vi "Begin.vi"(8 "error in":errorcluster) -> (0 "error out":errorcluster)   [LabVIEW 2018]
doc: "Called before other user functions, this VI can be used to open I/O refnums, load in file data, and do general program initialization. Notice that the <B>error out</B> terminal is simply used for data flow. Wiring it to other structures or subVIs ensures that this VI runs first."
uses:
  <vilib>/Rock Robotics/WPI/DriverStation/WPI_DriverStationRobotMode2.ctl
  <vilib>/Rock Robotics/WPI/Joystick/WPI_JoystickDeviceEnum.ctl
  <vilib>/Rock Robotics/SystemInterfaces/DIO/FPGA_DIOPWMChannel.ctl
  <vilib>/Rock Robotics/WPI/Solenoid/WPI_SolenoidChannel.ctl
  <vilib>/Rock Robotics/WPI/Solenoid/WPI_SolenoidValue.ctl
  <vilib>/Rock Robotics/WPI/SafetyOutput/WPI_SafetyOutputConfigMenu.ctl
  Robot Global Data.vi
  <vilib>/Rock Robotics/WPI/RobotDrive/WPI_RobotDriveOpen4MotorWithExistingMotors.vi
  <vilib>/Rock Robotics/WPI/RobotDrive/WPI_RobotDriveOpen2MotorWithExistingMotors.vi
  <vilib>/Rock Robotics/WPI/MotorControl/WPI_MotorControlOpen SPARK.vi
  <vilib>/Rock Robotics/WPI/Solenoid/WPI_SolenoidOpenDouble.vi
  <vilib>/Rock Robotics/WPI/Solenoid/WPI_SolenoidSetEnum.vi
panel:
  in  "Power Distribution Panel (0)":u8
  in  "Clear Sticky Faults":bool=TRUE
  out "Current Faults":bool[](array[boolean])
  out "Battery Voltage Fault":bool
  out "Temperature Fault":bool
  out "Hardware Fault":bool
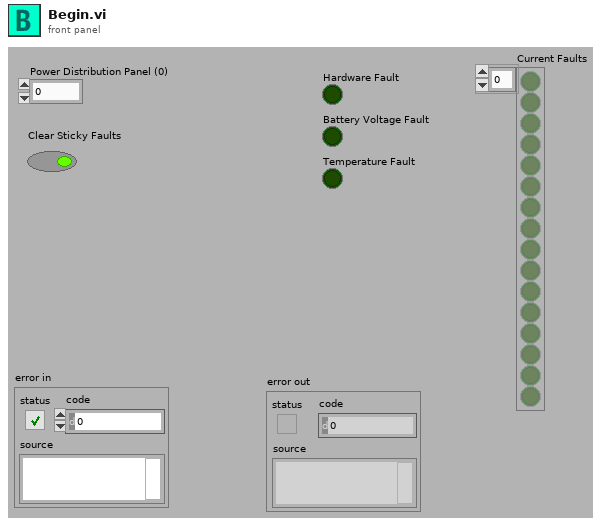
[diagram p1: front panel]
types:
  T1 = typedef "WPI_SafetyOutputConfigMenu.ctl" = enum16{"Enable", "Disable"}
  T2 = typedef "WPI_SolenoidValue.ctl" = enum16{"Off", "On", "Forward", "Reverse"}
  T3 = typedef "WPI_SolenoidChannel.ctl" = enum8{"Solenoid 0", "Solenoid 1", "Solenoid 2", "Solenoid 3", "Solenoid 4", "Solenoid 5", "Solenoid 6", "Solenoid 7", "Invalid"}
  T4 = typedef "FPGA_DIOPWMChannel.ctl" = enum8{"PWM 0", "PWM 1", "PWM 2", "PWM 3", "PWM 4", "PWM 5", "PWM 6", "PWM 7", "PWM 8", "PWM 9", "PWM MXP 0", "PWM MXP 1", "PWM MXP 2", "PWM MXP 3", "PWM MXP 4", "PWM MXP 5", "PWM MXP 6", "PWM MXP 7", "PWM MXP 8", "PWM MXP 9", "Invalid"}
  T5 = typedef "WPI_JoystickDeviceEnum.ctl" = enum16{"USB 0", "USB 1", "USB 2", "USB 3", "USB 4", "USB 5"}
  T6 = typedef "WPI_DriverStationRobotMode2.ctl" = enum16{"Autonomous Disabled", "Autonomous Enabled", "Teleop Disabled", "Teleop Enabled", "Disconnected", "Finish", "Test Disabled", "Test Enabled", "Emergency Stopped"}
  T7 = typedef "WPI_JoystickDevRef.ctl" = cluster{"Device":T5}
  T8 = typedef "WPI_MotorControlDeviceRef.ctl" = cluster{"DeviceStatus":errorcluster, "Type":T9, "PWM":cluster{"PWM Channel":T4, "DeadBand":T10}, "CAN":cluster{"Device Number":u8, "SetOutput VI Ref":variant, "GetOutput VI Ref":variant, "Enable VI Ref":variant, "Disable VI Ref":variant, "Data":variant}, "Invert":bool, "DIO PWM":cluster{"PWM \"Enable\" Channel":T4, "DIOChannel":T11, "PWM Rate":dbl}}
  T9 = typedef "WPI_MotorControlType.ctl" = enum16{"PWM", "CAN", "DIO PWM"}
  T10 = typedef "WPI_PWMDeadband.ctl" = cluster{"Name":string, "maxPositivePwm":i32, "minPositivePwm":i32, "centerPwm":i32, "maxNegativePwm":i32, "minNegativePwm":i32, "angularRange":u16}
  T11 = typedef "FPGA_DIOChannel.ctl" = enum8{"DIO 0", "DIO 1", "DIO 2", "DIO 3", "DIO 4", "DIO 5", "DIO 6", "DIO 7", "DIO 8", "DIO 9", "DIO MXP 0", "DIO MXP 1", "DIO MXP 2", "DIO MXP 3", "DIO MXP 4", "DIO MXP 5", "DIO MXP 6", "DIO MXP 7", "DIO MXP 8", "DIO MXP 9", "DIO MXP 10", "DIO MXP 11", "DIO MXP 12", "DIO MXP 13", "DIO MXP 14", "DIO MXP 15", "SPI Port CS1", "SPI Port CS2", "SPI Port CS3", "SPI Port MISO", "SPI Port MOSI", "Invalid"}
  T12 = typedef "WPI_RobotDriveDevRef.ctl" = cluster{"DevStatus":errorcluster, "Motors[]":T8[], "Square Inputs":bool, "Max Output":dbl}
  T13 = typedef "WPI_SolenoidDevRef.ctl" = cluster{"DevStatus":errorcluster, "Pneumatics Control Module":u8, "Forward Solenoid Channel":T3, "Reverse Solenoid Channel":T3}
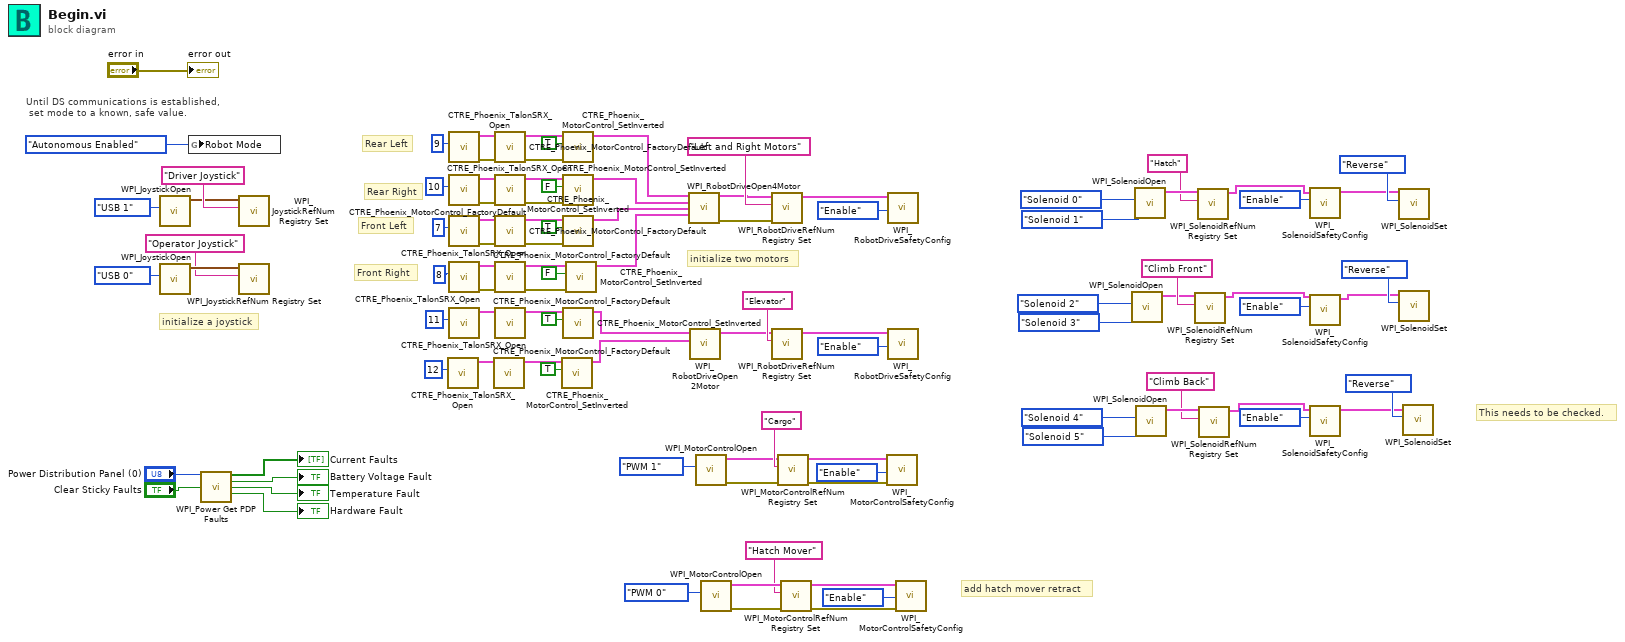
[diagram p0: block diagram]
diagram:
  # "This needs to be checked."
  # "add hatch mover retract"
  # "Front Right"
  # "Front Left"
  # "Rear Right"
  # "Rear Left"
  # "initialize two motors"
  # "initialize a joystick"
  # "Until DS communications is established,\n set mode to a known, safe value."
  n1 = call <vilib>:"WPI_JoystickOpen.vi"("JoystickDevice"=WPI_JoystickDeviceEnum."USB 1") -> ("JoystickDevRef"=w19:T7)  [unwired: 10 in]
  n2 = call <vilib>:"WPI_JoystickOpen.vi"("JoystickDevice"=WPI_JoystickDeviceEnum."USB 0") -> ("JoystickDevRef"=w16:T7)  [unwired: 10 in]
  n3 = global write "Robot Global Data.vi" "Robot Mode"(WPI_DriverStationRobotMode2."Autonomous Enabled" ("Robot Mode")) -> ()
  n4 = call <vilib>:"WPI_Power Get PDP Faults.vi"("Power Distribution Panel (0)"="Power Distribution Panel (0)", "Clear Sticky Faults"="Clear Sticky Faults") -> ("Current Faults"=→"Current Faults":bool[], "Battery Voltage Fault"=→"Battery Voltage Fault":bool, "Temperature Fault"=→"Temperature Fault":bool, "Hardware Fault"=→"Hardware Fault":bool)  [unwired: 9 in, 1 out]
  n5 = call <vilib>:"WPI_JoystickRefNum Registry Set.vi"("refnum name"="Driver Joystick", "JoystickDevRef"=w19) -> ()  [unwired: 8 in, 2 out]
  n6 = call <vilib>:"WPI_JoystickRefNum Registry Set.vi"("refnum name"="Operator Joystick", "JoystickDevRef"=w16) -> ()  [unwired: 8 in, 2 out]
  n7 = call <vilib>:"CTRE_Phoenix_TalonSRX_Open.vi"("Device Number"=u8 12) -> ("CAN Talon SRX Ref"=w56:T8)  [unwired: 9 in, 1 out]
  n8 = call <vilib>:"CTRE_Phoenix_TalonSRX_Open.vi"("Device Number"=u8 9) -> ("error out"=w38:errorcluster, "CAN Talon SRX Ref"=w39:T8)  [unwired: 9 in]
  n9 = call <vilib>:"CTRE_Phoenix_TalonSRX_Open.vi"("Device Number"=u8 10) -> ("error out"=w40:errorcluster, "CAN Talon SRX Ref"=w41:T8)  [unwired: 9 in]
  n10 = call <vilib>:"CTRE_Phoenix_TalonSRX_Open.vi"("Device Number"=u8 7) -> ("error out"=w42:errorcluster, "CAN Talon SRX Ref"=w43:T8)  [unwired: 9 in]
  n11 = call <vilib>:"CTRE_Phoenix_TalonSRX_Open.vi"("Device Number"=u8 8) -> ("error out"=w44:errorcluster, "CAN Talon SRX Ref"=w45:T8)  [unwired: 9 in]
  n12 = call <vilib>:"CTRE_Phoenix_TalonSRX_Open.vi"("Device Number"=u8 11) -> ("CAN Talon SRX Ref"=w59:T8)  [unwired: 9 in, 1 out]
  n13 = call <vilib>:"CTRE_Phoenix_MotorControl_FactoryDefault.vi"("PhoenixMotorControlDevRef"=w56) -> ("PhoenixMotorControlDevRef"=w57:T8)  [unwired: 9 in, 1 out]
  n14 = call <vilib>:"CTRE_Phoenix_MotorControl_FactoryDefault.vi"("error in"=w38, "PhoenixMotorControlDevRef"=w39) -> ("error out"=w47:errorcluster, "PhoenixMotorControlDevRef"=w46:T8)  [unwired: 8 in]
  n15 = call <vilib>:"CTRE_Phoenix_MotorControl_FactoryDefault.vi"("error in"=w40, "PhoenixMotorControlDevRef"=w41) -> ("error out"=w49:errorcluster, "PhoenixMotorControlDevRef"=w48:T8)  [unwired: 8 in]
  n16 = call <vilib>:"CTRE_Phoenix_MotorControl_FactoryDefault.vi"("error in"=w42, "PhoenixMotorControlDevRef"=w43) -> ("error out"=w51:errorcluster, "PhoenixMotorControlDevRef"=w50:T8)  [unwired: 8 in]
  n17 = call <vilib>:"CTRE_Phoenix_MotorControl_FactoryDefault.vi"("error in"=w44, "PhoenixMotorControlDevRef"=w45) -> ("error out"=w53:errorcluster, "PhoenixMotorControlDevRef"=w52:T8)  [unwired: 8 in]
  n18 = call <vilib>:"CTRE_Phoenix_MotorControl_FactoryDefault.vi"("PhoenixMotorControlDevRef"=w59) -> ("PhoenixMotorControlDevRef"=w58:T8)  [unwired: 9 in, 1 out]
  n19 = call <vilib>:"CTRE_Phoenix_MotorControl_SetInverted.vi"("Invert?"=TRUE, "PhoenixMotorControlDevRef"=w57) -> ("PhoenixMotorControlDevRef"=w77:T8)  [unwired: 8 in, 1 out]
  n20 = call <vilib>:"CTRE_Phoenix_MotorControl_SetInverted.vi"("error in (no error)"=w47, "Invert?"=TRUE, "PhoenixMotorControlDevRef"=w46) -> ("PhoenixMotorControlDevRef"=w37:T8)  [unwired: 7 in, 1 out]
  n21 = call <vilib>:"CTRE_Phoenix_MotorControl_SetInverted.vi"("error in (no error)"=w49, "Invert?"=FALSE, "PhoenixMotorControlDevRef"=w48) -> ("PhoenixMotorControlDevRef"=w32:T8)  [unwired: 7 in, 1 out]
  n22 = call <vilib>:"CTRE_Phoenix_MotorControl_SetInverted.vi"("error in (no error)"=w51, "Invert?"=TRUE, "PhoenixMotorControlDevRef"=w50) -> ("PhoenixMotorControlDevRef"=w35:T8)  [unwired: 7 in, 1 out]
  n23 = call <vilib>:"CTRE_Phoenix_MotorControl_SetInverted.vi"("Invert?"=TRUE, "PhoenixMotorControlDevRef"=w58) -> ("PhoenixMotorControlDevRef"=w76:T8)  [unwired: 8 in, 1 out]
  n24 = call <vilib>:"CTRE_Phoenix_MotorControl_SetInverted.vi"("error in (no error)"=w53, "Invert?"=FALSE, "PhoenixMotorControlDevRef"=w52) -> ("PhoenixMotorControlDevRef"=w30:T8)  [unwired: 7 in, 1 out]
  n25 = call-poly <vilib>:"WPI_RobotDriveOpen4Motor.vi"("Rear Left Motor Dev Ref"=w37, "Rear Right Motor Dev Ref"=w32, "Front Left Motor Dev Ref"=w35, "Front Right Motor Dev Ref"=w30) -> ("RobotDriveDevRef"=w21:T12, "error out"=w23:errorcluster)  [unwired: 10 in]
  n26 = call-poly <vilib>:"WPI_RobotDriveOpen2Motor.vi"("Right Motor Dev Ref"=w77, "Left Motor Dev Ref"=w76) -> ("RobotDriveDevRef"=w80:T12)  [unwired: 8 in, 1 out]
  n27 = call-poly <vilib>:"WPI_MotorControlOpen.vi"("PWM Channel"=FPGA_DIOPWMChannel."PWM 1") -> ("error out"=w62:errorcluster, "MotorControlDeviceRef"=w63:T8)  [unwired: 9 in]
  n28 = call-poly <vilib>:"WPI_MotorControlOpen.vi"("PWM Channel"=FPGA_DIOPWMChannel."PWM 0") -> ("error out"=w75:errorcluster, "MotorControlDeviceRef"=w74:T8)  [unwired: 9 in]
  n29 = call <vilib>:"WPI_RobotDriveRefNum Registry Set.vi"("error in (no error)"=w23, "refnum name"="Left and Right Motors", "RobotDriveDevRef"=w21) -> ("RobotDriveDevRef"=w24:T12)  [unwired: 1 in, 7 out]
  n30 = call <vilib>:"WPI_RobotDriveRefNum Registry Set.vi"("refnum name"="Elevator", "RobotDriveDevRef"=w80) -> ("RobotDriveDevRef"=w79:T12)  [unwired: 2 in, 7 out]
  n31 = call <vilib>:"WPI_MotorControlRefNum Registry Set.vi"("error in (no error)"=w62, "refnum name"="Cargo", "MotorControlDevRef"=w63) -> ("error out"=w64:errorcluster, "MotorControlDevRef"=w65:T8)  [unwired: 7 in]
  n32 = call <vilib>:"WPI_MotorControlRefNum Registry Set.vi"("error in (no error)"=w75, "refnum name"="Hatch Mover", "MotorControlDevRef"=w74) -> ("error out"=w73:errorcluster, "MotorControlDevRef"=w72:T8)  [unwired: 7 in]
  n33 = call <vilib>:"WPI_MotorControlSafetyConfig.vi"("error in (no error)"=w64, "mode"=WPI_SafetyOutputConfigMenu."Enable", "MotorControlDevRef"=w65) -> ()  [unwired: 7 in, 2 out]
  n34 = call <vilib>:"WPI_RobotDriveSafetyConfig.vi"("mode"=WPI_SafetyOutputConfigMenu."Enable", "RobotDriveDevRef"=w24) -> ()  [unwired: 8 in, 2 out]
  n35 = call <vilib>:"WPI_RobotDriveSafetyConfig.vi"("mode"=WPI_SafetyOutputConfigMenu."Enable", "RobotDriveDevRef"=w79) -> ()  [unwired: 8 in, 2 out]
  n36 = call <vilib>:"WPI_MotorControlSafetyConfig.vi"("error in (no error)"=w73, "mode"=WPI_SafetyOutputConfigMenu."Enable", "MotorControlDevRef"=w72) -> ()  [unwired: 7 in, 2 out]
  n37 = call-poly <vilib>:"WPI_SolenoidOpen.vi"("Reverse Solenoid Channel"=WPI_SolenoidChannel."Solenoid 3", "Forward Solenoid Channel"=WPI_SolenoidChannel."Solenoid 2" ("Solenoid Channel")) -> ("SolenoidDevRef"=w83:T13)  [unwired: 8 in, 1 out]
  n38 = call-poly <vilib>:"WPI_SolenoidOpen.vi"("Reverse Solenoid Channel"=WPI_SolenoidChannel."Solenoid 1", "Forward Solenoid Channel"=WPI_SolenoidChannel."Solenoid 0" ("Solenoid Channel")) -> ("SolenoidDevRef"=w86:T13)  [unwired: 8 in, 1 out]
  n39 = call-poly <vilib>:"WPI_SolenoidOpen.vi"("Reverse Solenoid Channel"=WPI_SolenoidChannel."Solenoid 5", "Forward Solenoid Channel"=WPI_SolenoidChannel."Solenoid 4" ("Solenoid Channel")) -> ("SolenoidDevRef"=w13:T13)  [unwired: 8 in, 1 out]
  n40 = call <vilib>:"WPI_SolenoidRefNum Registry Set.vi"("refnum name"="Climb Front", "SolenoidDevRef"=w83) -> ("SolenoidDevRef"=w4:T13)  [unwired: 8 in, 1 out]
  n41 = call <vilib>:"WPI_SolenoidRefNum Registry Set.vi"("refnum name"="Hatch", "SolenoidDevRef"=w86) -> ("SolenoidDevRef"=w6:T13)  [unwired: 8 in, 1 out]
  n42 = call <vilib>:"WPI_SolenoidRefNum Registry Set.vi"("refnum name"="Climb Back", "SolenoidDevRef"=w13) -> ("SolenoidDevRef"=w2:T13)  [unwired: 8 in, 1 out]
  n43 = call <vilib>:"WPI_SolenoidSafetyConfig.vi"("mode"=WPI_SafetyOutputConfigMenu."Enable", "SolenoidDevRef"=w6) -> ("SolenoidDevRef"=w5:T13)  [unwired: 8 in, 1 out]
  n44 = call <vilib>:"WPI_SolenoidSafetyConfig.vi"("mode"=WPI_SafetyOutputConfigMenu."Enable", "SolenoidDevRef"=w4) -> ("SolenoidDevRef"=w3:T13)  [unwired: 8 in, 1 out]
  n45 = call <vilib>:"WPI_SolenoidSafetyConfig.vi"("mode"=WPI_SafetyOutputConfigMenu."Enable", "SolenoidDevRef"=w2) -> ("SolenoidDevRef"=w1:T13)  [unwired: 8 in, 1 out]
  n46 = call-poly <vilib>:"WPI_SolenoidSet.vi"("Value"=WPI_SolenoidValue."Reverse", "SolenoidDevRef"=w5) -> ()  [unwired: 8 in, 2 out]
  n47 = call-poly <vilib>:"WPI_SolenoidSet.vi"("Value"=WPI_SolenoidValue."Reverse", "SolenoidDevRef"=w3) -> ()  [unwired: 8 in, 2 out]
  n48 = call-poly <vilib>:"WPI_SolenoidSet.vi"("Value"=WPI_SolenoidValue."Reverse", "SolenoidDevRef"=w1) -> ()  [unwired: 8 in, 2 out]
  "error out" <- "error in"
